vi "read allowed execution modes.vi"(8 "error in":errorcluster, 11 "Getting Started IO editor node in":refnum<class "UI Reference editor node.lvclass">) -> (0 "error out":errorcluster, 2 "allowed execution modes":T1[](array[typedef]), 3 "Getting Started IO editor node out":refnum<class "UI Reference editor node.lvclass">)   [LabVIEW 2013, in "UI Reference editor node.lvclass"]
uses:
  UI Reference editor node.lvclass
  <vilib>/NI/Tag Bus Data Framework/Configuration Editor/Classes/Module editor node/Allowed Execution Modes.ctl
  <vilib>/NI/Tag Bus Data Framework/Configuration Editor/Classes/Module editor node/module editor node.lvclass
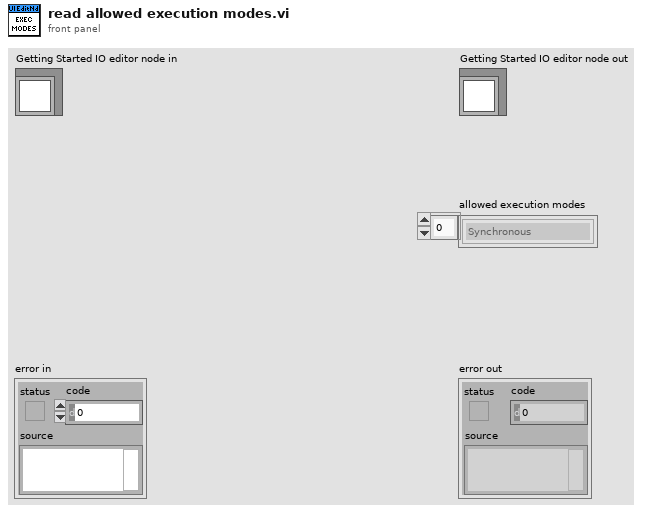
[diagram p1: front panel]
types:
  T1 = typedef "PL Framework Configuration Tool.lvlib/module editor node.lvclass/Allowed Execution Modes.ctl" = enum16{"Synchronous", "Asynchronous"}
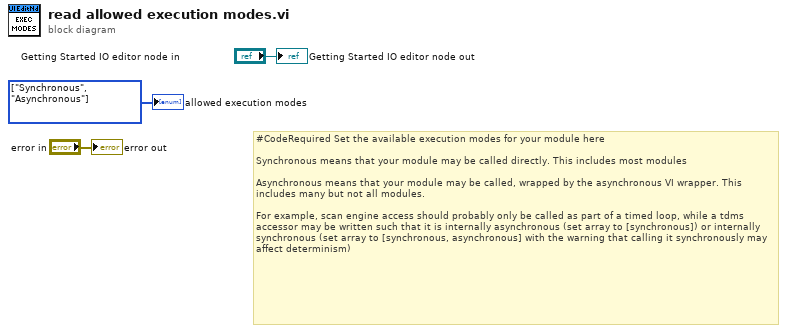
[diagram p0: block diagram]
diagram:
  w1 = T1[] [enum."Synchronous", enum."Asynchronous"] items=["Synchronous", "Asynchronous"] ("allowed execution modes")
  # "#CodeRequired Set the available execution modes for your module here\n\nSynchronous means that your module may be called directly. This includes most modules\n\nAsynchronous means that your module may be called, wrapped by the asynchronous VI wrapper. This includes many but not all modules. \n\nFor example, scan engine access should probably only be called as part of a timed loop, while a tdms accessor may be written such that it is internally asynchronous (set array to [synchronous]) or internally synchronous (set array to [synchronous, asynchronous] with the warning that calling it synchronously may affect determinism)"
  "error out" <- "error in"
  "Getting Started IO editor node out" <- "Getting Started IO editor node in"
  "allowed execution modes" <- w1
